vi "second.vi"() -> ()   [LabVIEW 2020]
uses:
  <vilib>/MakerHub/LINX/Public/Peripherals/Analog/Analog Read 1 Chan.vi
  <vilib>/MakerHub/LINX/Public/Peripherals/Digital/Digital Write 1 Chan.vi
  <vilib>/MakerHub/LINX/Public/Peripherals/Analog/Analog Read N Chans.vi
  <vilib>/MakerHub/LINX/Public/Peripherals/Digital/Digital Write N Chans.vi
  <vilib>/MakerHub/LINX/Private/Local IO/LinxAnalogRead.vi
  <vilib>/MakerHub/LINX/Public/Utilities/Check Channel.vi
  <vilib>/MakerHub/LINX/Private/Local IO/LinxDigitalWrite.vi
  <vilib>/MakerHub/LINX/Public/Utilities/Open Serial.vi
  <vilib>/MakerHub/LINX/Private/Utilties/Generate Error.vi
  <vilib>/MakerHub/LINX/LMH-LINX.lvlib
panel:
  in  "stop":bool
  out "Low":bool
  in  "High":dbl
  out "Status":string
  out "High":bool
  out "Normal":bool
  in  "Low":dbl
  out "Normal":dbl
  out "temperature":dbl(slide) scale=0.0..100.0
  out "Voltage":dbl(knob) scale=0.0..10.0
  in  "Analog Channel":u8
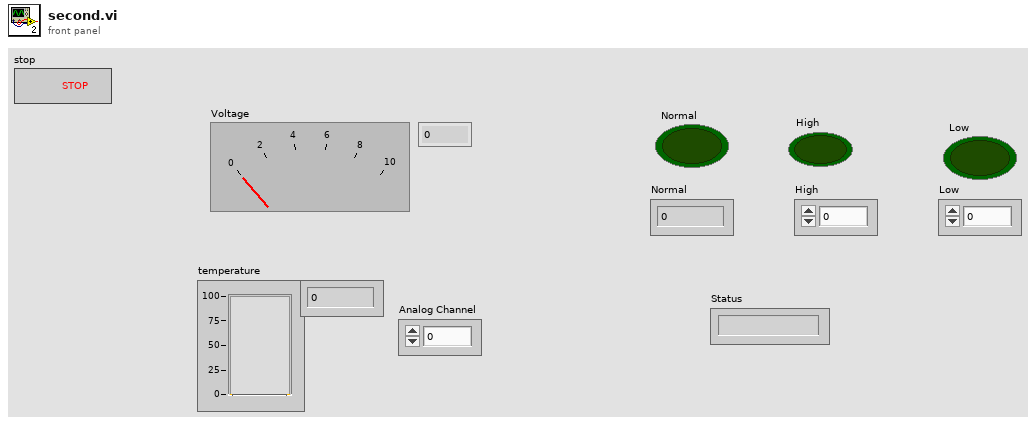
[diagram p1: front panel]
types:
  T1 = typedef "LMH-LINX.lvlib/LINX Ref.ctl" = cluster{"IO":T2, "Interface":T3, "LINX Device Config":T4}
  T2 = typedef "LMH-LINX.lvlib/Platform.ctl" = enum16{"Remote", "Local"}
  T3 = typedef "LMH-LINX.lvlib/Interface.ctl" = enum16{"Serial", "TCP"}
  T4 = typedef "LMH-LINX.lvlib/Device.lvlib/LINX Device Config.ctl" = cluster{"Interface":T3, "COM Port":refnum<visa-resource-name>, "TCP Configuration":T5, "Device Family":u8, "Device ID":u8, "Device Name":string, "TCP Ref":refnum<k5>, "Channels":T6}
  T5 = typedef "LMH-LINX.lvlib/Device.lvlib/TCP Config.ctl" = cluster{"IP Address":string, "Port":u16}
  T6 = typedef "LMH-LINX.lvlib/Channels.ctl" = cluster{"DI":u8[], "DO":u8[], "AI":u8[], "AO":u8[], "PWM":u8[], "QE":u8[], "UART":u8[], "I2C 2":u8[], "SPI":u8[], "CAN":u8[], "Servo":u8[], "AI Ref (V)":dbl, "AI Resolution (Bits)":u8, "AO Ref (V)":dbl, "AO Resolution (Bits)":u8}
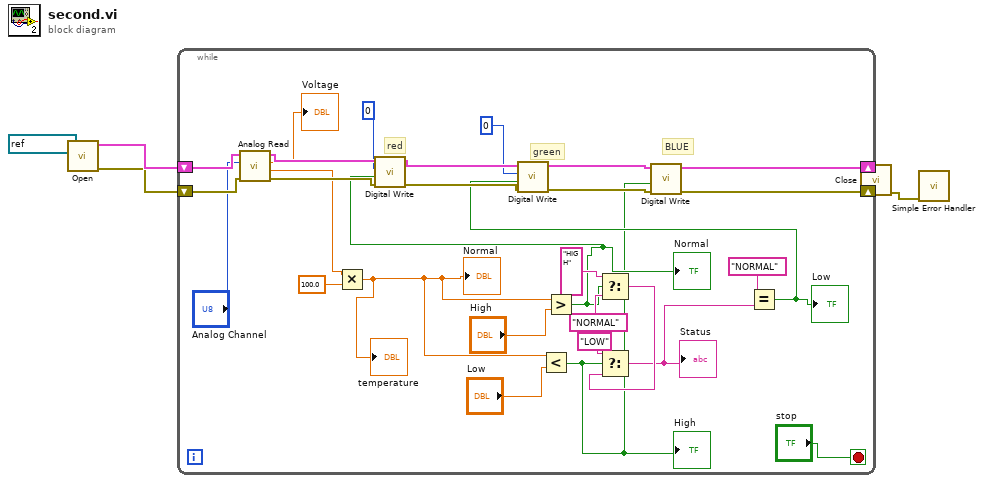
[diagram p0: block diagram]
diagram:
  n1 = call-poly <vilib>:"Open.vi"("Serial Port"=refnum<visa-resource-name> "COM14") -> ("Error Out"=w3:errorcluster, "LINX Resource"=w4:T1)  [unwired: 8 in, 1 out]
  n2 = while {
    shift-right: [w17] -> w5
    shift-left: w4 -> [w33]
    shift-right: [w16] -> w6
    shift-left: w3 -> [w32]
    stop <- "stop" stop-if-true
    # "BLUE"
    # "green"
    # "red"
    n3 = call-poly <vilib>:"Analog Read.vi"("Error In"=w32, "Analog Channel"="Analog Channel", "LINX Resource"=w33) -> ("Error Out"=w31:errorcluster, "AI Ref"=w24:dbl, "Voltage"=→"Voltage":dbl, "LINX Resource"=w34:T1)  [unwired: 5 in]
    n4 = Multiply(x=w24, y=100.0) -> (x*y=w21:dbl)
    "temperature" <- w21
    "Normal" <- w21
    n5 = Less?(x=w21, y="Low") -> (x < y?=w8:bool)
    "High" <- w8
    n6 = Greater?(x=w21, y="High") -> (0:w9:bool)
    "Normal" <- w9
    n7 = call-poly <vilib>:"Digital Write.vi"("Error In"=w31, "Output Value"=w9, "DO Channel"=u8 0, "LINX Resource"=w34) -> ("Error Out"=w30:errorcluster, "LINX Resource"=w35:T1)  [unwired: 6 in]
    n8 = Select(t="HIGH", s=w9, f="NORMAL") -> (s? t:f=w18:string)
    n9 = Select(t="LOW", s=w8, f=w18) -> (s? t:f=w11:string)
    "Status" <- w11
    n10 = Equal?(x="NORMAL", y=w11) -> (x = y?=w10:bool)
    "Low" <- w10
    n11 = call-poly <vilib>:"Digital Write.vi"("Error In"=w30, "Output Value"=w10, "DO Channel"=u8 0, "LINX Resource"=w35) -> ("Error Out"=w14:errorcluster, "LINX Resource"=w15:T1)  [unwired: 6 in]
    n12 = call-poly <vilib>:"Digital Write.vi"("Error In"=w14, "Output Value"=w8, "LINX Resource"=w15) -> ("Error Out"=w16:errorcluster, "LINX Resource"=w17:T1)  [unwired: 7 in]
  }
  n13 = call <vilib>:"Close.vi"("Error In"=w6, "LINX Resource"=w5) -> ("Error Out"=w2:errorcluster)  [unwired: 9 in]
  n14 = call <vilib>:"Simple Error Handler.vi"("error in (no error)"=w2) -> ()  [unwired: 4 in, 5 out]
